vi "getMasterRect.vi"(8 "error in (no error)":errorcluster, 11 "ref":refnum<vi>) -> (0 "error out":errorcluster, 2 "rect":T1, 3 "ref(dup)":refnum<vi>)   [LabVIEW 2023, in "TLC_Geometry.lvlib"]
uses:
  TLC_Geometry.lvlib
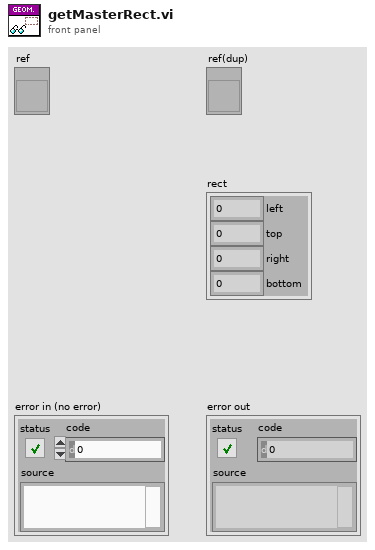
[diagram p1: front panel]
types:
  T1 = cluster{"left":i32, "top":i32, "right":i32, "bottom":i32}
  T2 = typedef "LVPositionTypeDef.ctl" = cluster{"Left":i32, "Top":i32}
  T3 = typedef "LVBoundsTypeDef.ctl" = cluster{"Width":u32, "Height":u32}
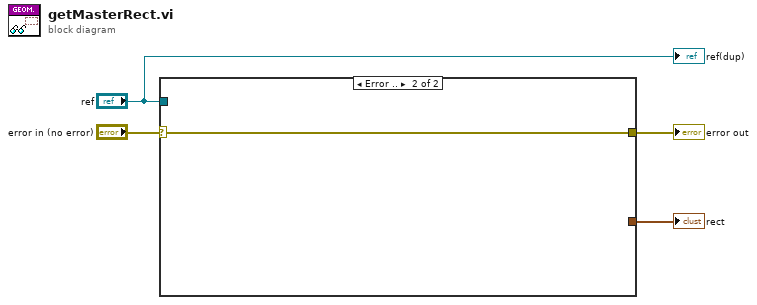
[diagram p0: block diagram]
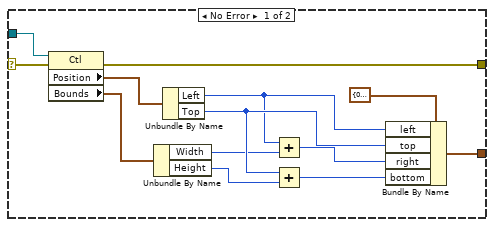
[diagram p2: hidden frame]
diagram:
  n1 = case shown="Error .." "error in (no error)" {
    selector: "error in (no error)" -> [w15 w18]
    tunnel: [w17 _] -> w4
    tunnel: [w16 w18] -> w3
    tunnel: "ref" -> [w5 _]
    frame No Error {
      n2 = property class="Ctl"(reference=w5, error in=w15) -> (error out=w16:errorcluster, "Position"=w7:T2, "Bounds"=w8:T3)  [unwired: 1 out]
      n3 = Unbundle By Name(w8) -> ("Width"=w10:u32, "Height"=w13:u32)
      n4 = Unbundle By Name(w7) -> ("Left"=w9:i32, "Top"=w12:i32)
      n5 = Add(x=w9, y=w10) -> (x+y=w11:u32)
      n6 = Add(x=w12, y=w13) -> (x+y=w14:u32)
      n7 = Bundle By Name(cluster=T1 {"left"=0, "top"=0, "right"=0, "bottom"=0} ("rect"), "left"=w9, "top"=w12, "right"=w11, "bottom"=w14) -> (w17:T1)
    }
    frame Error {
    }
  }
  "rect" <- w4
  "error out" <- w3
  "ref(dup)" <- "ref"
